vi "VISA Connection Read.vi"() -> ()   [LabVIEW 2014, in "VISA Connection Template.lvlib"]
uses:
  VISA Connection Template.lvlib
  <vilib>/Instr/_visa.llb/Select Event Type.ctl
panel:
  out "Buff out":string
  out "Error Out":errorcluster
  in  "Error In":errorcluster
  out "VISA out":refnum<visa-resource-name>
  in  "VISA in":refnum<visa-resource-name>
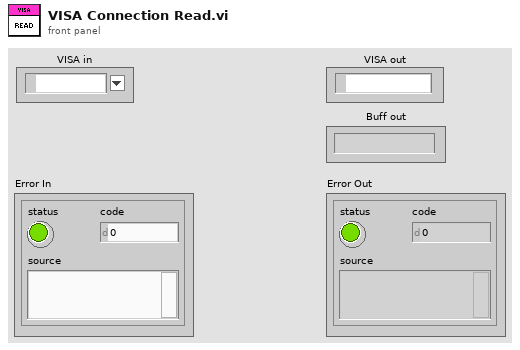
[diagram p1: front panel]
types:
  T1 = typedef "Select Event Type.ctl" = u32
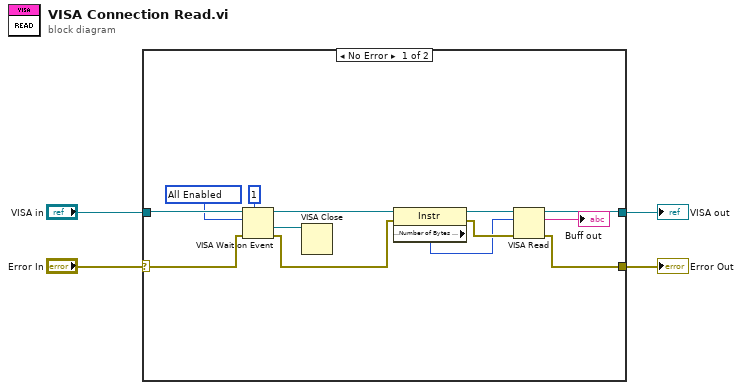
[diagram p0: block diagram]
diagram:
  n1 = case shown="No Error" "Error In" {
    selector: "Error In" -> [w14 w19]
    tunnel: [w7 w19] -> w3
    tunnel: "VISA in" -> [w17 w18]
    tunnel: [w12 w18] -> w1
    frame No Error {
      w15 = T1 1073709055 items=["Service Request"=1073684491, "Trigger"=3221168138, "Clear"=1073684493, "VXI Signal"=1073684512, "VXI/VME Interrupt"=3221168161, "VXI/VME Sysfail"=1073684509, "VXI/VME Sysreset"=1073684510, "GPIB CIC"=1073684498, "GPIB Talk"=1073684499, "GPIB Listen"=1073684500, "PXI Interrupt"=1073684514, "Serial Break"=1073684515, "Serial TermChar"=1073684516, "Serial CTS"=1073684521, "Serial DSR"=1073684522, "Serial DCD"=1073684524, "Serial RI"=1073684526, "Serial Character"=1073684533, "USB Interrupt"=1073684535, "All Enabled"=1073709055] ("Event Type")
      n2 = VISA Wait on Event(7:u32 1 ("timeout (0)"), 8:w14, 10:w15, 11:w17) -> (0:w9:errorcluster, 1:w13:refnum<visa-resource-name>, 3:w10:refnum<visa-resource-name>)  [unwired: 1 in, 1 out]
      n3 = VISA Close(VISA resource name=w13) -> ()  [unwired: 1 in, 1 out]
      n4 = property class="Instr"(reference=w10, error in=w9) -> (reference out=w11:refnum<visa-resource-name>, error out=w8:errorcluster, "Serial Settings:Number of Bytes at Serial Port"=w6:u32)
      n5 = VISA Read(VISA resource name=w11, byte count=w6, error in (no error)=w8) -> (VISA resource name out=w12:refnum<visa-resource-name>, read buffer=→"Buff out":string, error out=w7:errorcluster)  [unwired: 1 out]
    }
    frame Error {
    }
  }
  "VISA out" <- w1
  "Error Out" <- w3
